vi "Dictionary Update (by scalar value).vi"(7 "unlock dictionary? (FALSE)":bool, 8 "error in (no error)":errorcluster, 10 "key-value":T1, 11 "dictionary":T2) -> (0 "error out":errorcluster, 2 "created new?":bool, 3 "dictionary out":T2)   [LabVIEW 2009]
doc: "Updates a single value in the dictionary, referenced by the key.\n\n<B>unlock dictionary</B> will unlock a previously locked dictionary. Locking a dictionary is useful when the values of keys store compound data, which might be modified in multiple locations."
uses:
  Dictionary Object RefNum.ctl
  Dictionary Object RefNum - Enum.ctl
  Dictionary Key Value Pair Cluster.ctl
panel:
  # "Dictionary Update (by scalar value).vi\n\nUpdates a single value in the dictionary, referenced by the key.\n\nPlease visit http://www.OpenG.org to learn about the\nOpen Source LabVIEW software movement.\n\nNOTICE -- YOU MUST LEAVE THIS NOTICE IN PLACE.  PER THE TERMS OF THE LICENSE BELOW, YOU MAY SUBLICENSE THIS SOFTWARE \nIN ANY WAY THAT DOES NOT CONFLICT WITH THIS LICENSE.\n\n### BSD License (http://www.opensource.org/licenses/bsd-license.php) Begin ###\n \nCopyright (c) 2005, Jim Kring <jim@jimkring.com>\n\nAll rights reserved.\n\nRedistribution and use in source and binary forms, with or without modification, are permitted provided that the following conditions are met:\n\n    * Redistributions of source code must retain the above copyright notice, this list of conditions and the following disclaimer.\n    * Redistributions in binary form must reproduce the above copyright notice, this list of conditions and the following disclaimer in the \n       documentation and/or other materials provided with the distribution.\n    * Neither the name of SciWare, James Kring, Inc., nor the names of its contributors may be used to endorse or promote products derived \n       from this software without specific prior written permission.\n\nTHIS SOFTWARE IS PROVIDED BY THE COPYRIGHT HOLDERS AND CONTRIBUTORS \"AS IS\" AND ANY EXPRESS OR IMPLIED WARRANTIES, \nINCLUDING, BUT NOT LIMITED TO, THE IMPLIED WARRANTIES OF MERCHANTABILITY AND FITNESS FOR A PARTICULAR PURPOSE ARE \nDISCLAIMED. IN NO EVENT SHALL THE COPYRIGHT OWNER OR CONTRIBUTORS BE LIABLE FOR ANY DIRECT, INDIRECT, INCIDENTAL,\n SPECIAL, EXEMPLARY, OR CONSEQUENTIAL DAMAGES (INCLUDING, BUT NOT LIMITED TO, PROCUREMENT OF SUBSTITUTE GOODS OR \nSERVICES; LOSS OF USE, DATA, OR PROFITS; OR BUSINESS INTERRUPTION) HOWEVER CAUSED AND ON ANY THEORY OF LIABILITY, \nWHETHER IN CONTRACT, STRICT LIABILITY, OR TORT (INCLUDING NEGLIGENCE OR OTHERWISE) ARISING IN ANY WAY OUT OF THE USE \nOF THIS SOFTWARE, EVEN IF ADVISED OF THE POSSIBILITY OF SUCH DAMAGE.\n\n### BSD License End ###"
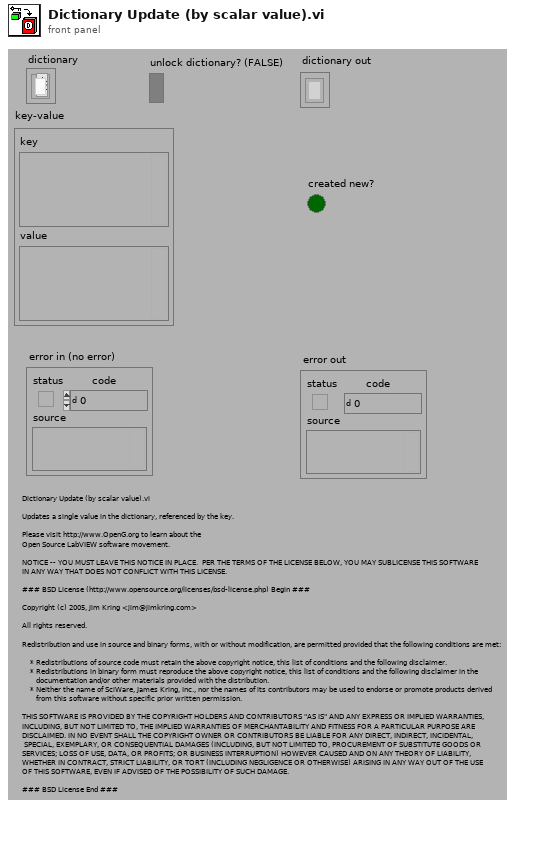
[diagram p1: front panel]
types:
  T1 = typedef "Dictionary Key Value Pair Cluster.ctl" = cluster{"key":variant, "value":variant}
  T2 = typedef "Dictionary Object RefNum.ctl" = refnum<k1>
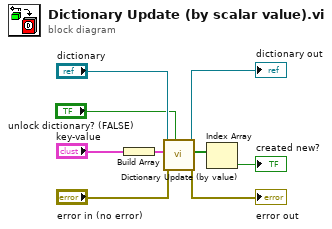
[diagram p0: block diagram]
diagram:
  n1 = Build Array("key-value") -> (w4:T1[])
  n2 = call "Dictionary Update (by value).vi"("unlock dictionary? (FALSE)"="unlock dictionary? (FALSE)", "error in (no error)"="error in (no error)", "dictionary with updates"=w4, "dictionary"="dictionary") -> ("error out"=→"error out":errorcluster, "created new?"=w3:bool[], "dictionary out"=→"dictionary out":T2)  [unwired: 5 in]
  n3 = Index Array(array=w3) -> (element=→"created new?":bool)  [unwired: 1 in]
